vi "Release.vi"(8 "error in (no error)":errorcluster, 11 "SingleB in":refnum<class "SingleB.lvclass">) -> (0 "error out":errorcluster, 3 "SingleB out":refnum<class "SingleB.lvclass">)   [LabVIEW 2020, in "SingleB.lvclass"]
uses:
  SingleB.lvclass
  Singleton/Singleton.lvclass
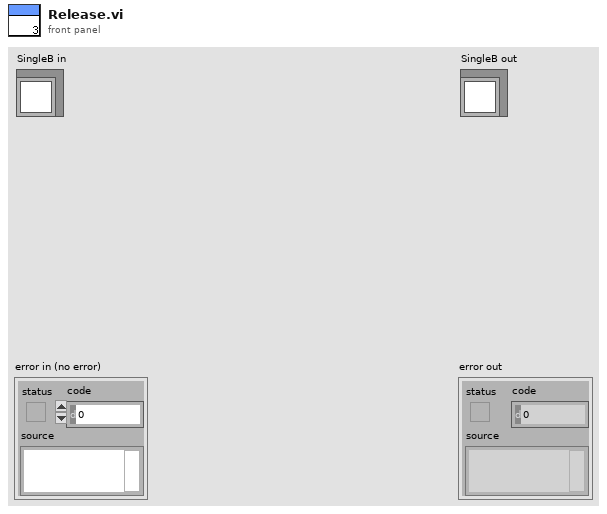
[diagram p1: front panel]
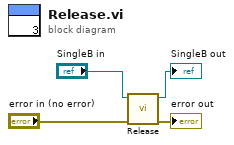
[diagram p0: block diagram]
diagram:
  n1 = call-parent "Release.vi"("error in (no error)"="error in (no error)", "Singleton in"="SingleB in") -> ("error out"=→"error out":errorcluster, "Singleton out"=→"SingleB out":refnum<class "SingleB.lvclass">)  [unwired: 8 in]
